vi "Extensometria1.vi"() -> ()   [LabVIEW 2017]
panel:
  out "DADO TENSÃO EXTENSOMETRO 8":dynamicdata(graph)
  out "DADO TENSÃO EXTENSOMETRO 7":dynamicdata(graph)
  out "DADO TENSÃO EXTENSOMETRO 6":dynamicdata(graph)
  out "DADO TENSÃO EXTENSOMETRO 5":dynamicdata(graph)
  out "DADO TENSÃO EXTENSOMETRO 4":dynamicdata(graph)
  out "DADO TENSÃO EXTENSOMETRO 3":dynamicdata(graph)
  out "DADO TENSÃO EXTENSOMETRO 2":dynamicdata(graph)
  out "DADO TENSÃO EXTENSOMETRO 1":dynamicdata(graph)
  out "DADO FILTRADO EXTENSOMETRO 8":dynamicdata(graph)
  out "DADO FILTRADO EXTENSOMETRO 7":dynamicdata(graph)
  out "DADO FILTRADO EXTENSOMETRO 6":dynamicdata(graph)
  out "DADO FILTRADO EXTENSOMETRO 5":dynamicdata(graph)
  out "DADO FILTRADO EXTENSOMETRO 4":dynamicdata(graph)
  out "DADO FILTRADO EXTENSOMETRO 3":dynamicdata(graph)
  out "DADO FILTRADO EXTENSOMETRO 2":dynamicdata(graph)
  out "DADO FILTRADO EXTENSOMETRO 1":dynamicdata(graph)
  out "DADO BRUTO EXTENSOMETRO 8":dynamicdata(graph)
  out "DADO BRUTO EXTENSOMETRO 7":dynamicdata(graph)
  out "DADO BRUTO EXTENSOMETRO 6":dynamicdata(graph)
  out "DADO BRUTO EXTENSOMETRO 5":dynamicdata(graph)
  out "DADO BRUTO EXTENSOMETRO 4":dynamicdata(graph)
  out "DADO BRUTO EXTENSOMETRO 3":dynamicdata(graph)
  out "DADO BRUTO EXTENSOMETRO 2":dynamicdata(graph)
  out "DADO BRUTO EXTENSOMETRO 1":dynamicdata(graph)
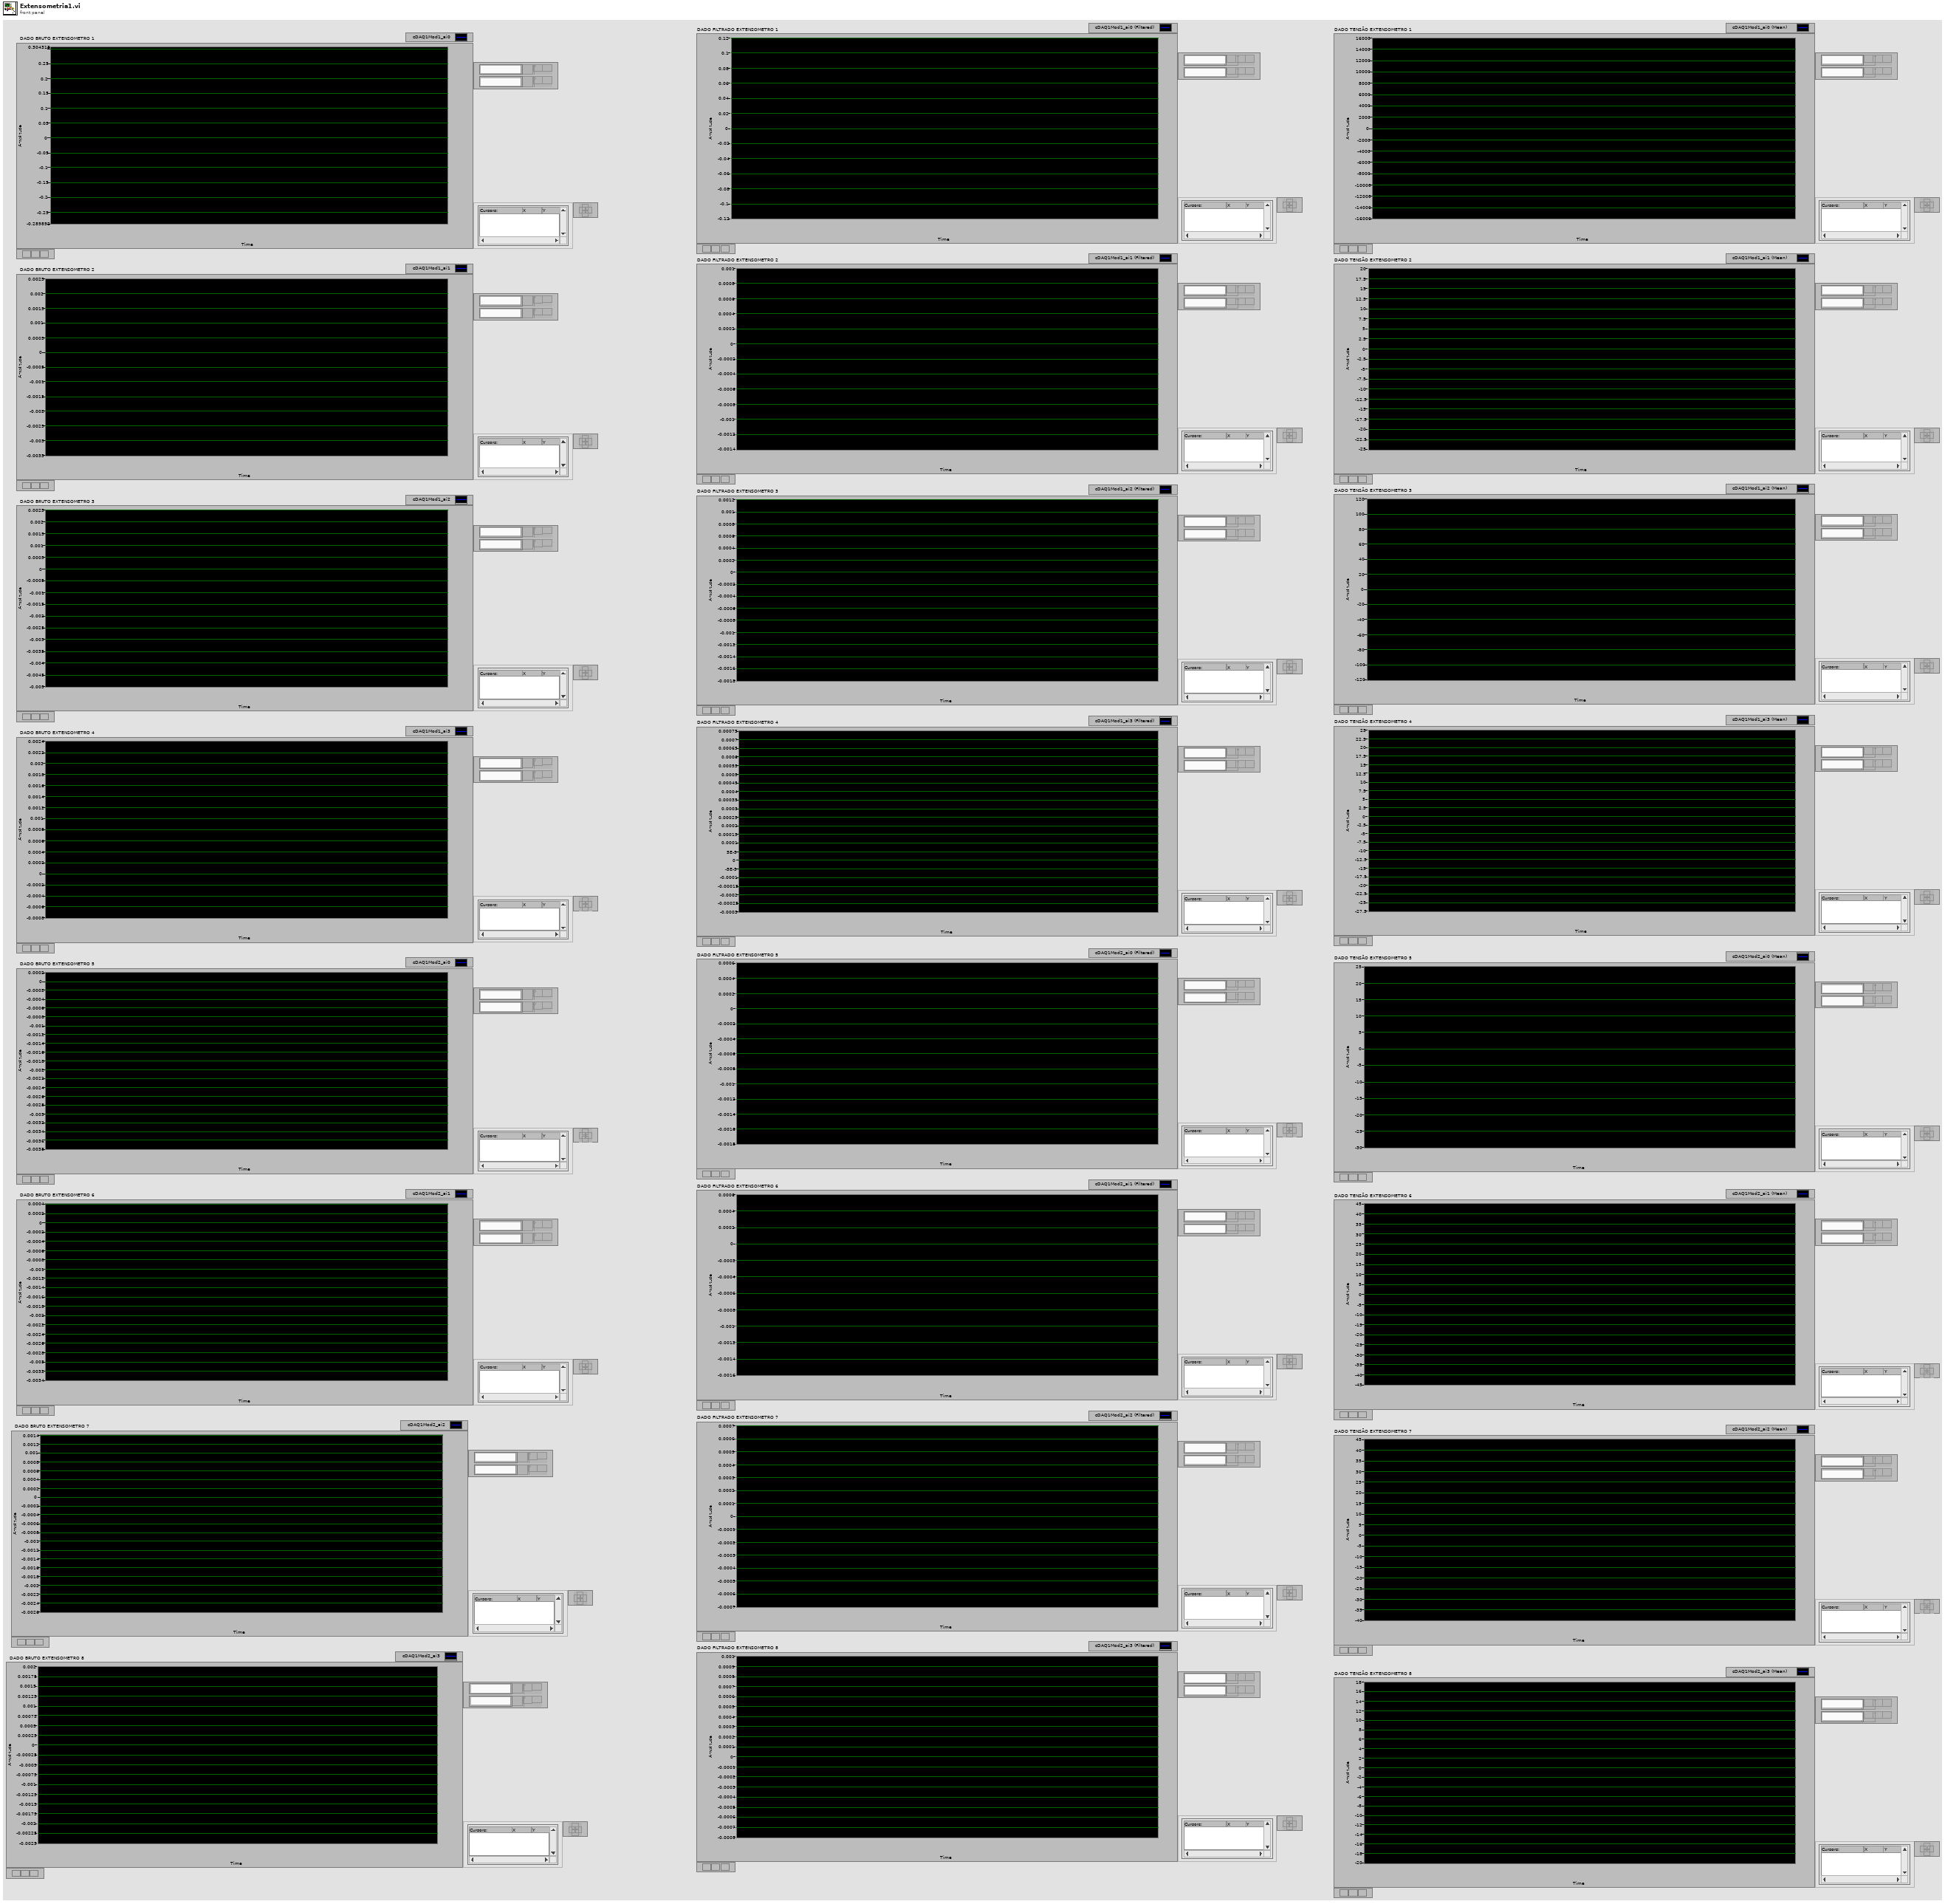
[diagram p1: front panel]
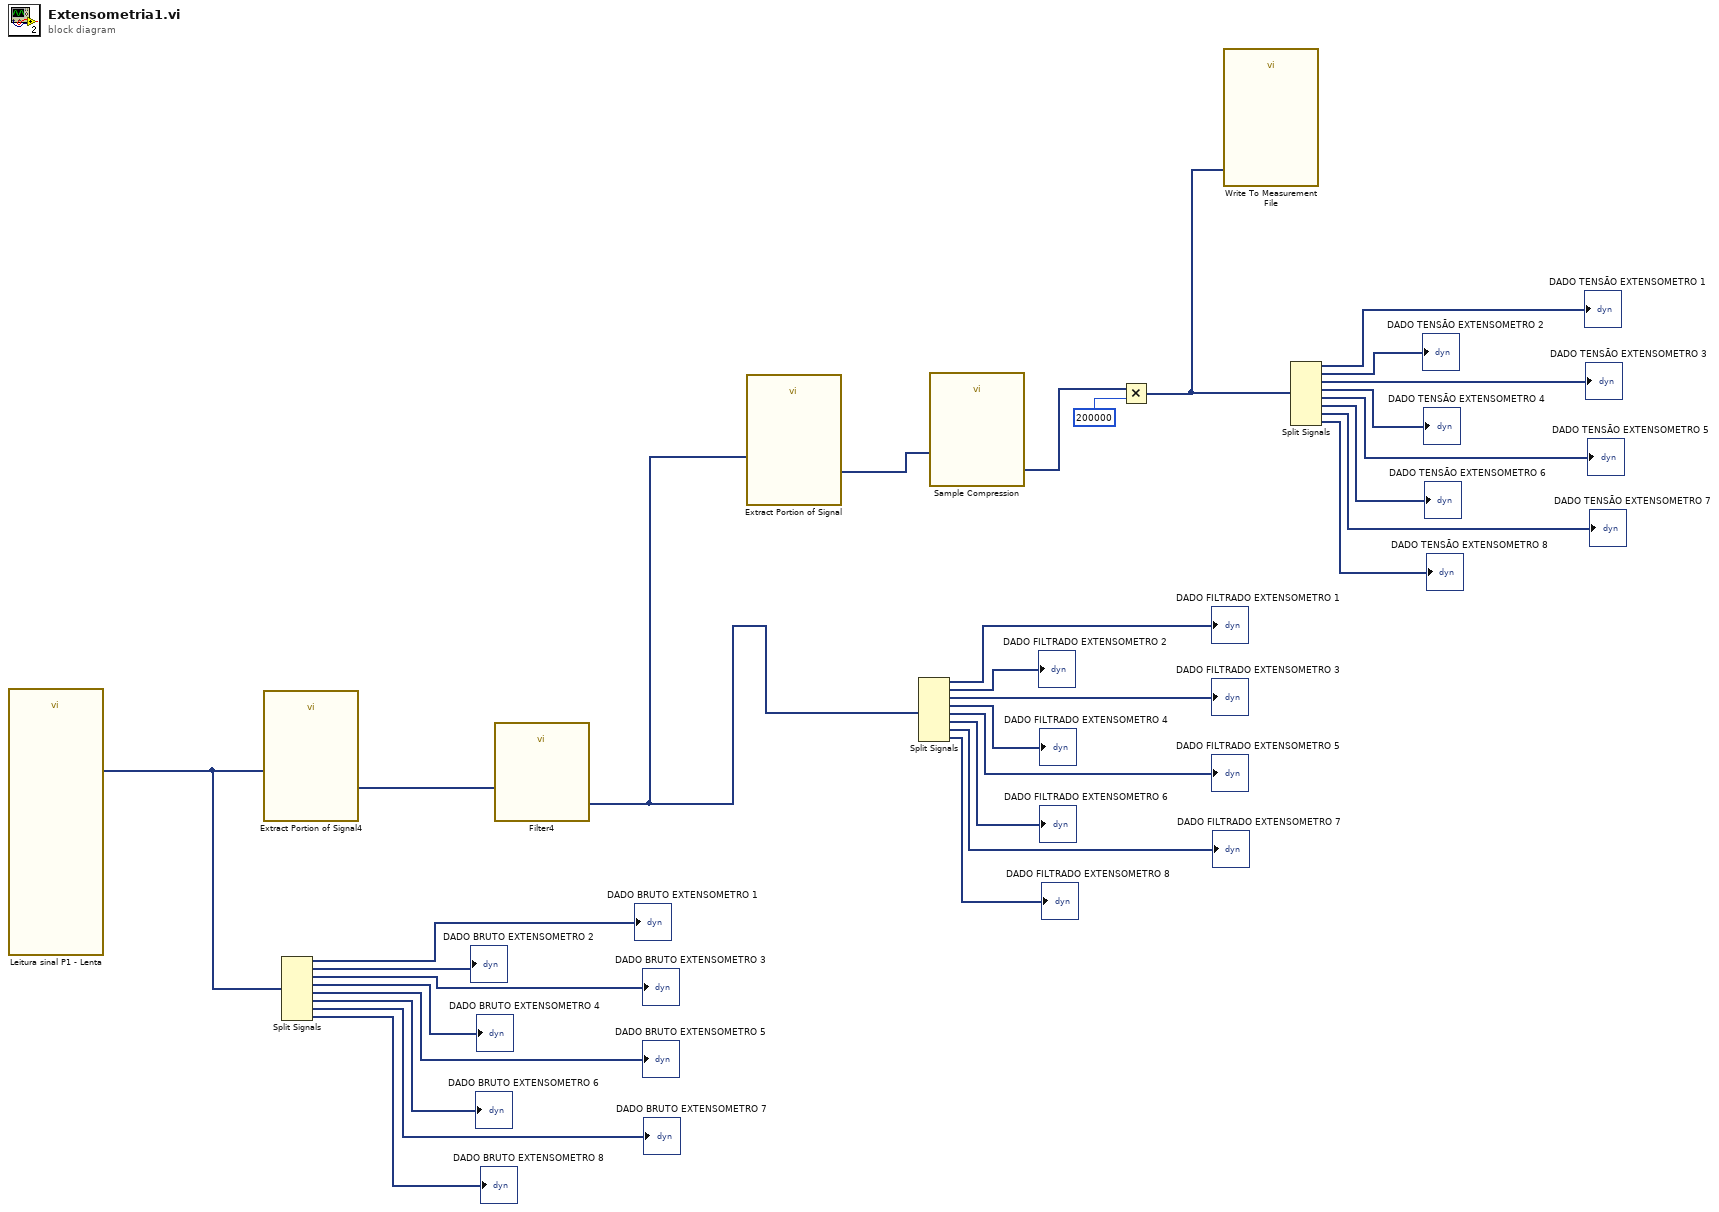
[diagram p0: block diagram]
diagram:
  n1 = call "Leitura sinal P1 - Lenta"() -> ("Signals"=w30:dynamicdata)  [unwired: 6 in, 5 out]
  n2 = call "Extract Portion of Signal4"("Signals"=w30) -> ("Section"=w31:dynamicdata)  [unwired: 9 in, 1 out]
  n3 = Split Signals(w30) -> (→"DADO BRUTO EXTENSOMETRO 1":dynamicdata, →"DADO BRUTO EXTENSOMETRO 2":dynamicdata, →"DADO BRUTO EXTENSOMETRO 3":dynamicdata, →"DADO BRUTO EXTENSOMETRO 4":dynamicdata, →"DADO BRUTO EXTENSOMETRO 5":dynamicdata, →"DADO BRUTO EXTENSOMETRO 6":dynamicdata, →"DADO BRUTO EXTENSOMETRO 7":dynamicdata, →"DADO BRUTO EXTENSOMETRO 8":dynamicdata)  [unwired: 8 in]
  n4 = call "Filter4"("Signal"=w31) -> ("Filtered Signal"=w11:dynamicdata)  [unwired: 9 in, 1 out]
  n5 = call "Extract Portion of Signal"("Signals"=w11) -> ("Section"=w10:dynamicdata)  [unwired: 9 in, 1 out]
  n6 = Split Signals(w11) -> (→"DADO FILTRADO EXTENSOMETRO 1":dynamicdata, →"DADO FILTRADO EXTENSOMETRO 2":dynamicdata, →"DADO FILTRADO EXTENSOMETRO 3":dynamicdata, →"DADO FILTRADO EXTENSOMETRO 4":dynamicdata, →"DADO FILTRADO EXTENSOMETRO 5":dynamicdata, →"DADO FILTRADO EXTENSOMETRO 6":dynamicdata, →"DADO FILTRADO EXTENSOMETRO 7":dynamicdata, →"DADO FILTRADO EXTENSOMETRO 8":dynamicdata)  [unwired: 8 in]
  n7 = call "Sample Compression"("Signals"=w10) -> ("Mean"=w12:dynamicdata)  [unwired: 8 in, 2 out]
  n8 = Multiply(x=w12, y=200000) -> (x*y=w9:dynamicdata)
  n9 = call "Write To Measurement File"("Signals"=w9) -> ()  [unwired: 16 in, 3 out]
  n10 = Split Signals(w9) -> (→"DADO TENSÃO EXTENSOMETRO 1":dynamicdata, →"DADO TENSÃO EXTENSOMETRO 2":dynamicdata, →"DADO TENSÃO EXTENSOMETRO 3":dynamicdata, →"DADO TENSÃO EXTENSOMETRO 4":dynamicdata, →"DADO TENSÃO EXTENSOMETRO 5":dynamicdata, →"DADO TENSÃO EXTENSOMETRO 6":dynamicdata, →"DADO TENSÃO EXTENSOMETRO 7":dynamicdata, →"DADO TENSÃO EXTENSOMETRO 8":dynamicdata)  [unwired: 8 in]
